vi "Save Offset Angle to File.vi"(8 "error in (no error)":errorcluster, 10 "servo ID (0)":i32, 11 "ccw offset angle (rad)":dbl) -> (0 "error out":errorcluster, 1 "failed?":bool, 3 "coerced ccw offset angle (rad)":dbl)   [LabVIEW 2017, in "NI_Robotics_Starter Kit Servo Motor.lvclass"]
uses:
  <vilib>/robotics/Starter Kit/Servo Motor/NI_Robotics_Starter Kit Servo Motor.lvclass
  <vilib>/Utility/file.llb/Dflt Data Dir.vi
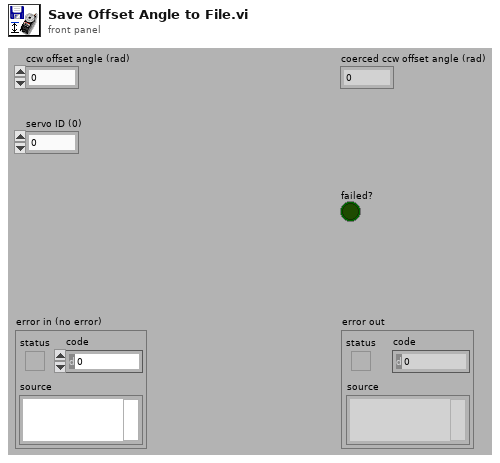
[diagram p1: front panel]
types:
  T1 = enum16{"open", "replace", "create", "open or create", "replace or create", "replace or create with confirmation"}
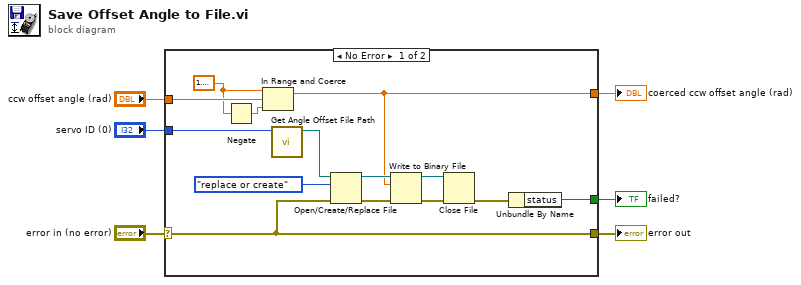
[diagram p0: block diagram]
diagram:
  n1 = case shown="No Error" "error in (no error)" {
    selector: "error in (no error)" -> [w11 w22]
    tunnel: [w11 w22] -> w4
    tunnel: "ccw offset angle (rad)" -> [w10 w21]
    tunnel: [w14 _] -> w3
    tunnel: "servo ID (0)" -> [w13 _]
    tunnel: [w7 w21] -> w1
    frame No Error {
      w8 = 1.5707963267948966
      n2 = Negate(x=w8) -> (-x=w9:dbl)
      n3 = In Range and Coerce(upper limit=w8, x=w10, lower limit=w9) -> (coerced(x)=w7:dbl)  [unwired: 1 out]
      n4 = call <vilib>:"Get Angle Offset File Path.vi"("servo ID (0)"=w13) -> ("angle offset file path"=w12:path)  [unwired: 10 in]
      n5 = Open/Create/Replace File(file path (use dialog)=w12, error in=w11, operation (0:open)=T1."replace or create") -> (refnum out=w16:refnum<file>, error out=w17:errorcluster)  [unwired: 3 in, 1 out]
      n6 = Write to Binary File(file (use dialog)=w16, data=w7, error in=w17) -> (refnum out=w18:refnum<file>, error out=w19:errorcluster)  [unwired: 3 in, 1 out]
      n7 = Close File(refnum=w18, error in=w19) -> (error out=w20:errorcluster)  [unwired: 1 out]
      n8 = Unbundle By Name(w20) -> ("status"=w14:bool)
    }
    frame Error {
    }
  }
  "failed?" <- w3
  "error out" <- w4
  "coerced ccw offset angle (rad)" <- w1
